vi "Single DI.vi"() -> ()   [LabVIEW 2023, in "CTI-Visa-Scratchpad.lvlib"]
uses:
  CTI-Visa-Scratchpad.lvlib
  CTI-Visa/Digital Direction.ctl
  CTI-Visa/Digital Pull Direction.ctl
  CTI-Visa/CTI-Visa.lvlib
panel:
  out "Readback":bool
  in  "Port":refnum<visa-resource-name>="COM3"
  in  "stop":bool
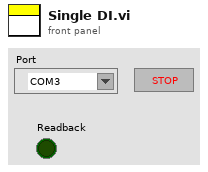
[diagram p1: front panel]
types:
  T1 = typedef "CTI-Visa.lvlib/Digital Pull Direction.ctl" = enum16{"None", "Up", "Down", "Both"}
  T2 = typedef "CTI-Visa.lvlib/Digital Direction.ctl" = enum16{"In", "Out"}
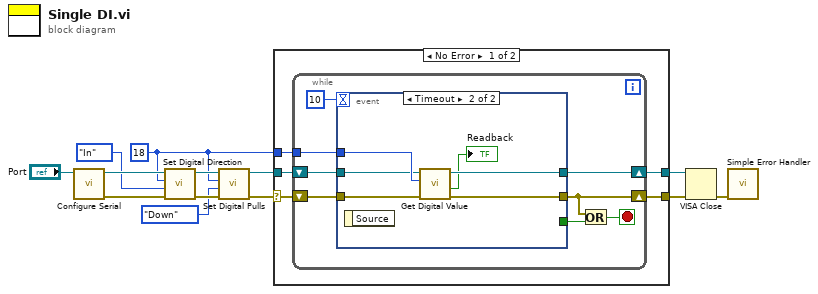
[diagram p0: block diagram]
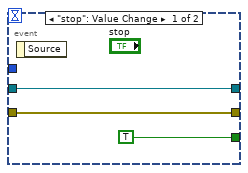
[diagram p2: hidden frame]
diagram:
  w2 = 18 ("Channel")
  n1 = call "Configure Serial.vi"("VISA resource name in"="Port") -> ("error out"=w11:errorcluster, "VISA resource name"=w12:refnum<visa-resource-name>)  [unwired: 9 in]
  n2 = call "Set Digital Direction.vi"("error in (no error)"=w11, "Direction"=Digital_Direction."In", "Channel"=w2, "VISA resource name in"=w12) -> ("error out"=w10:errorcluster, "VISA resource name"=w4:refnum<visa-resource-name>)  [unwired: 6 in]
  n3 = call "Set Digital Pulls.vi"("error in (no error)"=w10, "Pull"=Digital_Pull_Direction."Down", "Channel"=w2, "VISA resource name in"=w4) -> ("error out"=w5:errorcluster, "VISA resource name"=w3:refnum<visa-resource-name>)  [unwired: 6 in]
  n4 = case shown="No Error" w5 {
    selector: w5 -> [w17 w36]
    tunnel: w3 -> [w18 w37]
    tunnel: [w16 w37] -> w9
    tunnel: [w15 w36] -> w8
    tunnel: w2 -> [w14 _]
    frame No Error {
      n5 = while {
        shift-right: [w24] -> w16
        shift-left: w18 -> [w26]
        shift-right: [w23] -> w15
        shift-left: w17 -> [w25]
        tunnel: w14 -> [w20]
        stop <- w22 stop-if-true
        n6 = event shown="[1] Timeout" {
          selector: _ -> [_ _]
          dyn-events: _ -> [_ _]
          timeout: 10 -> [_ _]
          tunnel: w26 -> [w29 w31]
          tunnel: w25 -> [w28 w30]
          tunnel: [w29 w35] -> w24
          tunnel: [w28 w34] -> w23
          tunnel: [TRUE _] -> w21
          tunnel: w20 -> [_ w32]
          event "stop": Value Change {
            n7 = event-data() -> ()  [unwired: 1 in, 1 out]
          }
          event Timeout {
            n8 = event-data() -> ()  [unwired: 1 in, 1 out]
            n9 = call "Get Digital Value.vi"("error in (no error)"=w30, "Channel"=w32, "VISA resource name in"=w31) -> ("error out"=w34:errorcluster, "Value"=→"Readback":bool, "VISA resource name"=w35:refnum<visa-resource-name>)  [unwired: 6 in]
          }
        }
        n10 = Or(x=w23, y=w21) -> (x .or. y?=w22:bool)
      }
    }
    frame Error {
    }
  }
  n11 = VISA Close(VISA resource name=w9, error in (no error)=w8) -> (error out=w7:errorcluster)
  n12 = call <vilib>:"Simple Error Handler.vi"("error in (no error)"=w7) -> ()  [unwired: 4 in, 5 out]
